vi "TDMS Delete Group.vi"(8 "error in (no error)":errorcluster, 9 "File Path In":path, 10 "Run to Delete":i32, 11 "TDMS File Ref":refnum<k34>) -> (0 "error out":errorcluster, 1 "File Path Out":path, 2 "Run #":i32, 3 "TDMS File Ref":refnum<k34>)   [LabVIEW 2011]
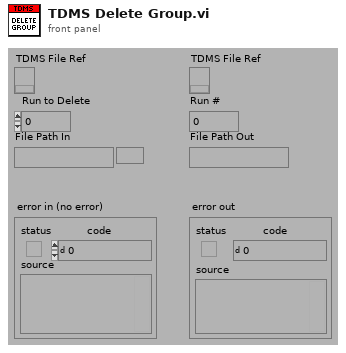
[diagram p1: front panel]
types:
  T1 = enum16{"open", "open or create", "create or replace", "create", "open (read-only)"}
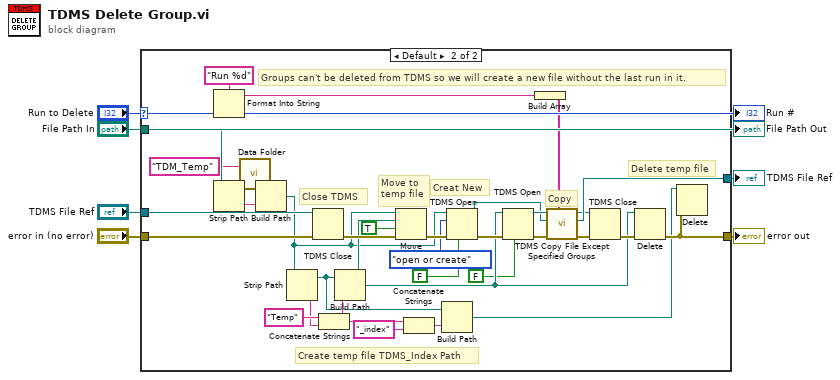
[diagram p0: block diagram]
diagram:
  n1 = case shown="Default" "Run to Delete" {
    selector: "Run to Delete" -> [_ w10]
    tunnel: "TDMS File Ref" -> [w7 w38]
    tunnel: [w8 w37] -> w5
    tunnel: [w7 w36] -> w4
    tunnel: "error in (no error)" -> [w8 w26]
    tunnel: "File Path In" -> [_ w13]
    frame ..0 {
      # "Not a valid run to delete."
    }
    frame Default {
      # "Groups can't be deleted from TDMS so we will create a new file without the last run in it."
      # "Create temp file TDMS_Index Path"
      # "Delete temp file"
      # "Copy"
      # "Creat New"
      # "Move to\ntemp file"
      # "Close TDMS"
      n2 = Format Into String(format string="Run %d", w10) -> (resulting string=w19:string)  [unwired: 2 in, 1 out]
      n3 = Strip Path(path=w13) -> (name=w14:string)  [unwired: 1 out]
      n4 = call "Data Folder.vi"("Relative Path (\"\" - Folder)"="TDM_Temp" ("Relative Path (\"\" - Folder)")) -> ("Data Folder"=w15:path)  [unwired: 2 in]
      n5 = Build Path(base path=w15, name or relative path=w14) -> (appended path=w25:path)
      n6 = Strip Path(path=w25) -> (stripped path=w16:path, name=w17:string)
      n7 = TDMS Close(8:w26, 11:w38) -> (0:w41:errorcluster)  [unwired: 1 out]
      n8 = Concatenate Strings("Temp" ("string"), w17) -> (w30:string)
      n9 = Build Path(base path=w16, name or relative path=w30) -> (appended path=w31:path)
      n10 = Move(source path=w25, error in=w41, 9:TRUE ("overwrite (F)"), 10:w31) -> (error out=w35:errorcluster)  [unwired: 3 out]
      n11 = Concatenate Strings(w30, "_index" ("string")) -> (w28:string)
      n12 = Build Path(base path=w16, name or relative path=w28) -> (appended path=w27:path)
      n13 = TDMS Open(6:FALSE ("disable buffering (T)"), 8:w35, 10:T1."open or create" ("operation (0:open)"), 11:w25) -> (0:w34:errorcluster, 3:w18:refnum<k34>)  [unwired: 2 in]
      n14 = TDMS Open(6:FALSE ("disable buffering (T)"), 8:w34, 11:w31) -> (0:w24:errorcluster, 3:w22:refnum<k34>)  [unwired: 3 in]
      n15 = Build Array(w19) -> (w20:string[])
      n16 = call "TDMS Copy File Except Specified Groups.vi"("Groups Names"=w20, "error in (no error)"=w24, "TDMS Destination In"=w18, "TDMS Source In"=w22) -> ("error out"=w23:errorcluster, "TDMS Destination Out"=w36:refnum<k34>, "TDMS Source Out"=w21:refnum<k34>)  [unwired: 5 out]
      n17 = TDMS Close(8:w23, 11:w21) -> (0:w32:errorcluster)  [unwired: 1 out]
      n18 = Delete(path (use dialog)=w31, error in=w32) -> (error out=w37:errorcluster)  [unwired: 5 out]
      n19 = Delete(path (use dialog)=w27, error in=w37) -> ()  [unwired: 6 out]
    }
  }
  "TDMS File Ref" <- w4
  "error out" <- w5
  "File Path Out" <- "File Path In"
  "Run #" <- "Run to Delete"
